vi "ADIS16448_RoboRIO_Teensy_Loop.vi"(8 "error in":errorcluster, 11 "SerialPortRef":T1) -> ()   [LabVIEW 2016, in "RoboRIO-Teensy-ADIS16448-Interface.lvlib"]
uses:
  RoboRIO-Teensy-ADIS16448-Interface.lvlib
  <vilib>/Rock Robotics/WPI/SerialPort/WPI_SerialPortRef.ctl
panel:
  out "Parsed Serial Data":dbl[](array[numeric])
  out "Raw Serial Data":string
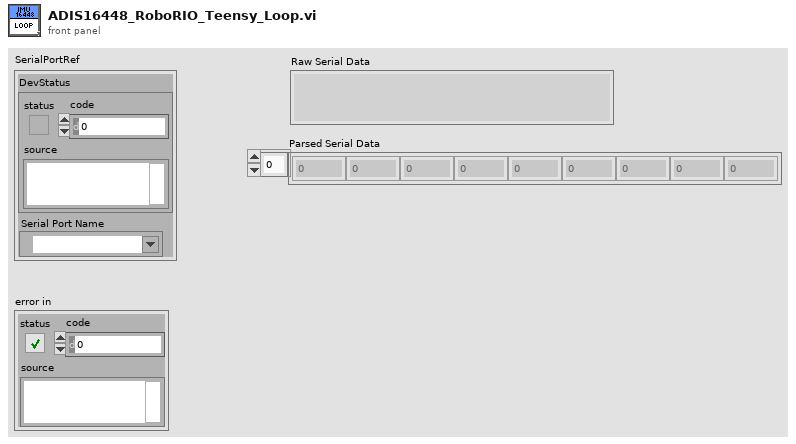
[diagram p1: front panel]
types:
  T1 = typedef "WPI_SerialPortRef.ctl" = cluster{"DevStatus":errorcluster, "Serial Port Name":refnum<visa-resource-name>}
  T2 = cluster{"X Angle":dbl, "Y Angle":dbl, "Z Angle":dbl}
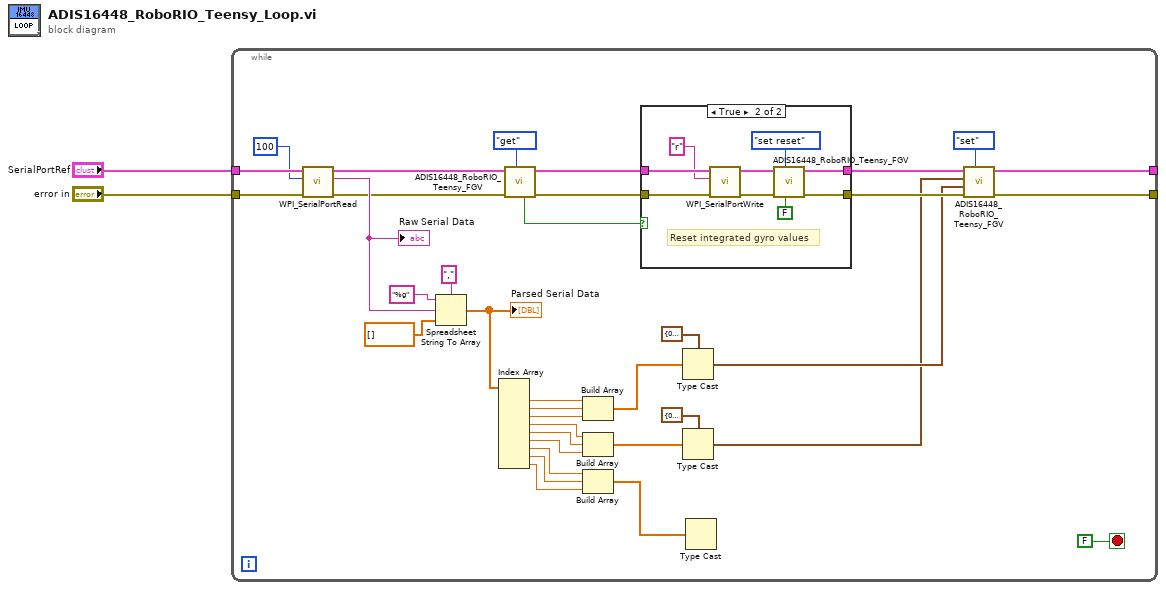
[diagram p0: block diagram]
diagram:
  n1 = while {
    tunnel: "SerialPortRef" -> [w38]
    tunnel: "error in" -> [w37]
    tunnel: [w22] -> _
    tunnel: [w21] -> _
    stop <- FALSE stop-if-true
    n2 = call <vilib>:"WPI_SerialPortRead.vi"("error in (no error)"=w37, "Num Bytes to Read"=u32 100, "SerialPortRef"=w38) -> ("error out"=w25:errorcluster, "Buffer"=w32:string, "SerialPortRef"=w29:T1)  [unwired: 6 in]
    "Raw Serial Data" <- w32
    n3 = Spreadsheet String To Array(delimiter (Tab)="," ("delimiter"), format string="%g", spreadsheet string=w32, array type (2D Dbl)=dbl[] []) -> (array=w19:dbl[])
    "Parsed Serial Data" <- w19
    n4 = Index Array(array=w19) -> (element #1=w18:dbl, element #2=w17:dbl, element #3=w16:dbl, element #4=w14:dbl, element #5=w13:dbl, element #6=w12:dbl, element #7=w5:dbl, element #8=w4:dbl, element #9=w6:dbl)  [unwired: 9 in]
    n5 = call "ADIS16448_RoboRIO_Teensy_FGV.vi"("Operation"=enum16{"set", "get", "set reset"}."get", "error in"=w25, "SerialPortRefIn"=w29) -> ("error out"=w26:errorcluster, "SerialPortRefOut"=w27:T1, "Reset Out"=w28:bool)  [unwired: 4 in, 2 out]
    n6 = Build Array(w18, w17, w16) -> (w15:dbl[])
    n7 = Build Array(w14, w13, w12) -> (w11:dbl[])
    n8 = Build Array(w5, w4, w6) -> (w3:dbl[])
    n9 = case shown="True" w28 {
      tunnel: w27 -> [w40 w49]
      tunnel: w26 -> [w39 w48]
      tunnel: [w40 w44] -> w24
      tunnel: [w39 w43] -> w23
      frame False {
      }
      frame True {
        # "Reset integrated gyro values"
        n10 = call <vilib>:"WPI_SerialPortWrite.vi"("error in (no error)"=w48, "Buffer"="r", "SerialPortRef"=w49) -> ("error out"=w42:errorcluster, "SerialPortRef"=w41:T1)  [unwired: 6 in, 1 out]
        n11 = call "ADIS16448_RoboRIO_Teensy_FGV.vi"("Reset"=FALSE, "Operation"=enum16{"set", "get", "set reset"}."set reset", "error in"=w42, "SerialPortRefIn"=w41) -> ("error out"=w43:errorcluster, "SerialPortRefOut"=w44:T1)  [unwired: 3 in, 3 out]
      }
    }
    n12 = Type Cast(type=cluster{"Pitch":dbl, "Roll":dbl, "Yaw":dbl} {"Pitch"=0.0, "Roll"=0.0, "Yaw"=0.0} ("IMU AHRS"), x=w15) -> (*(type *) &x=w8:cluster{"Pitch":dbl, "Roll":dbl, "Yaw":dbl})
    n13 = Type Cast(type=T2 {"X Angle"=0.0, "Y Angle"=0.0, "Z Angle"=0.0} ("IMU Angles"), x=w11) -> (*(type *) &x=w7:T2)
    n14 = Type Cast(x=w3) -> ()  [unwired: 1 in, 1 out]
    n15 = call "ADIS16448_RoboRIO_Teensy_FGV.vi"("Operation"=enum16{"set", "get", "set reset"}."set", "error in"=w23, "IMU AHRS"=w8, "IMU Angles"=w7, "SerialPortRefIn"=w24) -> ("error out"=w21:errorcluster, "SerialPortRefOut"=w22:T1)  [unwired: 2 in, 3 out]
  }
